vi "Z_Measurement.vi"(8 "error in (no error)":errorcluster, 10 "QuWire in":refnum<class "QuWire.lvclass">, 11 "SimAlg in":refnum<class "PrllPerElmnt.lvclass">) -> (0 "error out":errorcluster, 1 "Classical bit":bool, 2 "QuWire out":refnum<class "QuWire.lvclass">, 3 "SimAlg out":refnum<class "PrllPerElmnt.lvclass">)   [LabVIEW 2020, in "PrllPerElmnt.lvclass"]
uses:
  PrllPerElmnt.lvclass
  QuWire/QuWire.lvclass
  PrllPerElmnt.lvclass/PrllPerElmnt.ctl
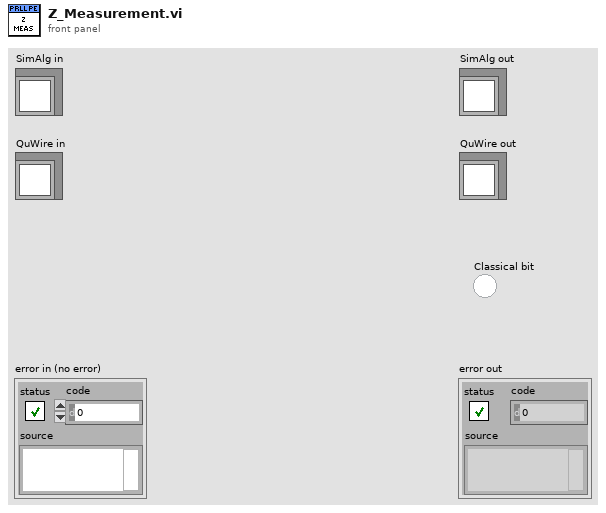
[diagram p1: front panel]
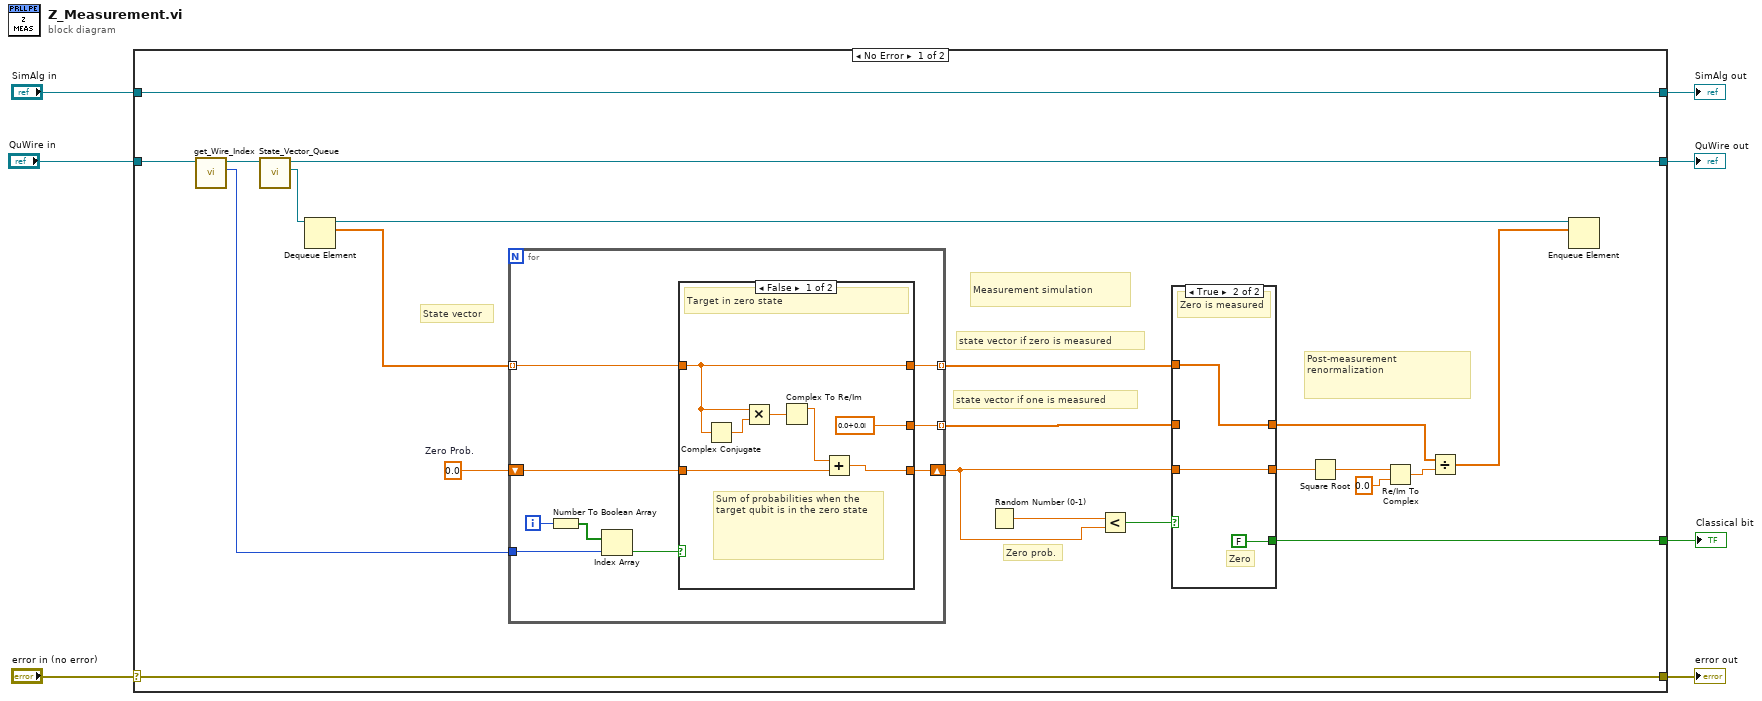
[diagram p0: block diagram]
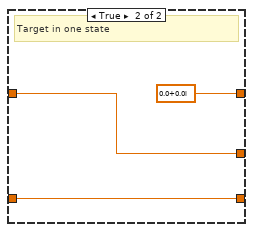
[diagram p2: hidden frame]
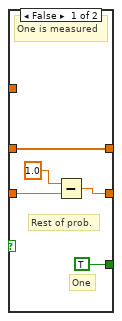
[diagram p3: hidden frame]
diagram:
  n1 = case shown="No Error" "error in (no error)" {
    selector: "error in (no error)" -> [w28 w59]
    tunnel: [w28 w59] -> w6
    tunnel: [w29 w58] -> w4
    tunnel: "SimAlg in" -> [w29 w58]
    tunnel: [w13 _] -> w3
    tunnel: "QuWire in" -> [w12 w57]
    tunnel: [w11 w57] -> w1
    frame No Error {
      w26 = 0.0  # Zero Prob.
      # "Zero prob."
      # "state vector if one is measured"
      # "state vector if zero is measured"
      # "State vector"
      # "Measurement simulation"
      # "Post-measurement renormalization"
      n2 = call "get_Wire_Index.vi"("QuWire in"=w12) -> ("Wire Index"=w16:i32, "QuWire out"=w17:refnum<class "QuWire.lvclass">)  [unwired: 8 in, 1 out]
      n3 = call "State_Vector_Queue.vi"("QuWire in"=w17) -> ("State Vector Queue"=w18:refnum<queue>, "QuWire out"=w11:refnum<class "QuWire.lvclass">)  [unwired: 8 in, 1 out]
      n4 = Dequeue Element(queue=w18) -> (queue out=w14:refnum<queue>, element=w15:cdb[])  [unwired: 2 in, 2 out]
      n5 = for {
        tunnel: w16 -> [w36]
        shift-right: [w33] -> w23
        shift-left: w26 -> [w34]
        tunnel: w15 -> [w32] mode=indexing
        tunnel: [w31] -> w22 mode=indexing
        tunnel: [w30] -> w21 mode=indexing
        i -> [w38]
        n6 = Number To Boolean Array(number=w38) -> (Boolean array=w37:bool[])
        n7 = Index Array "Index Array"(array=w37, index=w36) -> (element=w35:bool)
        n8 = case shown="False" w35 {
          tunnel: w34 -> [w45 w48]
          tunnel: [w44 w48] -> w33
          tunnel: w32 -> [w40 w47]
          tunnel: [w40 cdb 0.0+0.0i ("Complex Matrix Element")] -> w31
          tunnel: [cdb 0.0+0.0i ("Complex Matrix Element") w47] -> w30
          frame False {
            # "Sum of probabilities when the target qubit is in the zero state"
            # "Target in zero state"
            n9 = Complex Conjugate(1:w40) -> (0:w42:cdb)
            n10 = Multiply ("Multiply.vi")(x=w40, y=w42) -> (x*y=w41:cdb)
            n11 = Complex To Re/Im ("Complex To Cartesian.vi")(x + iy=w41) -> (x=w39:dbl)  [unwired: 1 out]
            n12 = Add(x=w39, y=w45) -> (x+y=w44:dbl)
          }
          frame True {
            # "Target in one state"
          }
        }
      }
      n13 = Random Number (0-1)() -> (number: 0 to 1=w25:dbl)
      n14 = Less?(x=w25, y=w23) -> (x < y?=w24:bool)
      n15 = case shown="True" w24 {
        tunnel: w23 -> [w53 w56]
        tunnel: w22 -> [_ w55]
        tunnel: w21 -> [w50 _]
        tunnel: [w51 w56] -> w20
        tunnel: [w50 w55] -> w19
        tunnel: [TRUE FALSE] -> w13
        frame False {
          # "One"
          # "Rest of prob."
          # "One is measured"
          n16 = Subtract(x=1.0, y=w53) -> (x-y=w51:dbl)
        }
        frame True {
          # "Zero"
          # "Zero is measured"
        }
      }
      n17 = Square Root(x=w20) -> (sqrt(x)=w8:dbl)
      n18 = Re/Im To Complex(1:0.0 ("y"), 2:w8) -> (0:w9:cdb)
      n19 = Divide(x=w19, y=w9) -> (x/y=w27:cdb[])
      n20 = Enqueue Element(queue=w14, element=w27) -> ()  [unwired: 2 in, 3 out]
    }
    frame Error {
    }
  }
  "error out" <- w6
  "SimAlg out" <- w4
  "QuWire out" <- w1
  "Classical bit" <- w3
